vi "CagingCalculator.vi"(11 "Calculate":bool) -> (3 "Position Array":cluster{"X Position":dbl, "Y Position":dbl}[](array[cluster])=[{"X Position"=0.0005, "Y Position"=0.00043}, {"X Position"=0.00055, "Y Position"=0.0005700000000000001}, {"X Position"=0.00045, "Y Position"=0.0005700000000000001}])   [LabVIEW 2014]
panel:
  out "Y Array":dbl[](array[numeric])
  out "X Array":dbl[](array[numeric])
  in  "Bubble radius":dbl
  in  "Y coordinate of object":dbl
  in  "X coordinate of object":dbl
  in  "Vertical radius":dbl
  in  "Horizontal radius":dbl
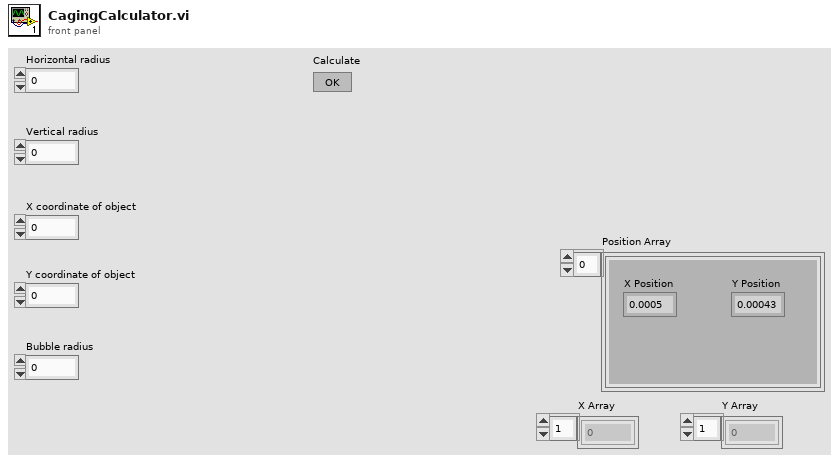
[diagram p1: front panel]
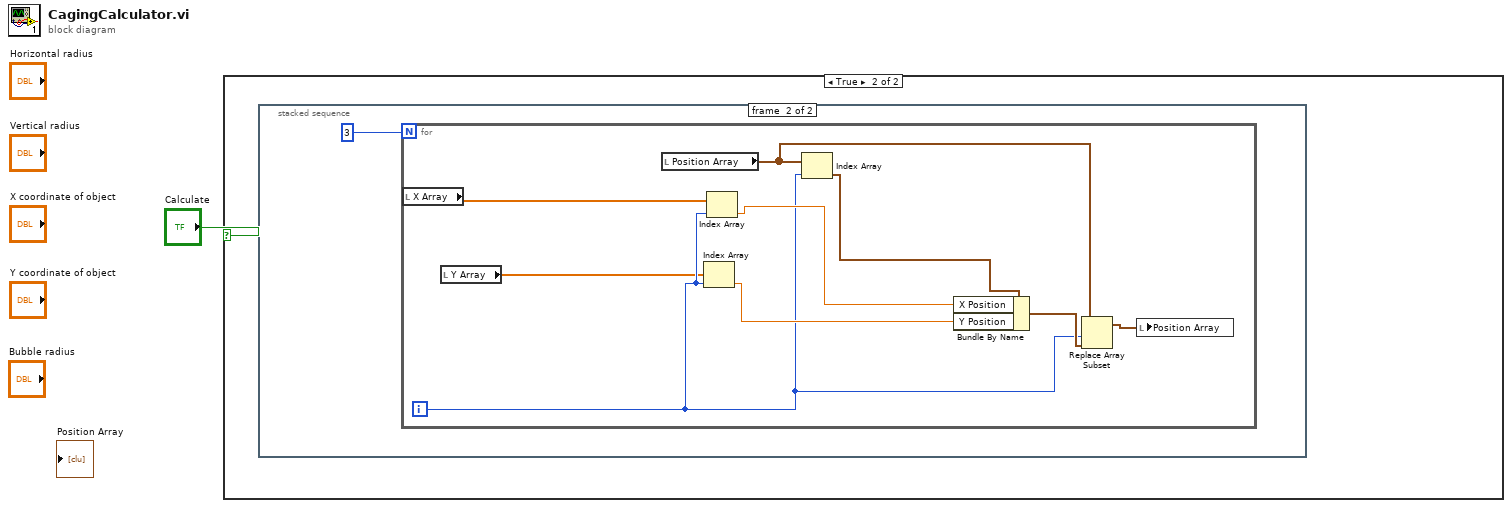
[diagram p0: block diagram]
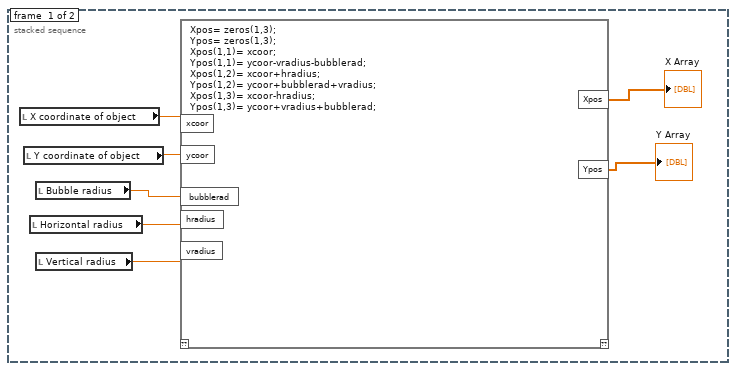
[diagram p3: hidden frame]
diagram:
  n1 = case shown="True" "Calculate" {
    frame False {
    }
    frame True {
      n2 = stacked-sequence {
        frame #0 {
          n3 = local read "X coordinate of object"() -> (w6:dbl)
          n4 = local read "Y coordinate of object"() -> (w5:dbl)
          n5 = local read "Horizontal radius"() -> (w3:dbl)
          n6 = local read "Bubble radius"() -> (w4:dbl)
          n7 = local read "Vertical radius"() -> (w2:dbl)
          n8 = script code="Xpos= zeros(1,3);\nYpos= zeros(1,3);\nXpos(1,1)= xcoor;\nYpos(1,1)= ycoor-vradius-bubblerad;\nXpos(1,2)= xcoor+hradius;\nYpos(1,2)= ycoor+bubblerad+vradius;\nXpos(1,3)= xcoor-hradius;\nYpos(1,3)= ycoor+vradius+bubblerad;"("xcoor"=w6, "ycoor"=w5, "bubblerad"=w4, "hradius"=w3, "vradius"=w2) -> ("Xpos"=→"X Array":dbl[], "Ypos"=→"Y Array":dbl[])  [unwired: 1 in, 1 out]
        }
        frame #1 {
          n9 = for {
            N: 3 -> [_]
            i -> [w12]
            n10 = local read "X Array"() -> (w11:dbl[])
            n11 = local read "Y Array"() -> (w10:dbl[])
            n12 = local read "Position Array"() -> (w16:cluster{"X Position":dbl, "Y Position":dbl}[])
            n13 = Index Array(array=w10, index=w12) -> (element=w14:dbl)
            n14 = Index Array(array=w11, index=w12) -> (element=w13:dbl)
            n15 = Index Array(array=w16, index=w12) -> (element=w18:cluster{"X Position":dbl, "Y Position":dbl})
            n16 = Bundle By Name(cluster=w18, "X Position"=w13, "Y Position"=w14) -> (w17:cluster{"X Position":dbl, "Y Position":dbl})
            n17 = Replace Array Subset(array=w16, new element=w17, index=w12) -> (w15:cluster{"X Position":dbl, "Y Position":dbl}[])
            n18 = local write "Position Array"(w15) -> ()
          }
        }
      }
    }
  }
